vi "Transfer Count (Plugin).vi"(8 "error in (no error)":errorcluster, 11 "Plugin Configuration in":T1={"name"="", "components"=[], "cycle timing"={"priority"=0, "decimation"=1, "offset"=0}, "threads"=[], "Transfer Groups"=[], "settings"=[]} {"Transfer Groups"."Transfers"."channels"."string offset" format="%d bytes"}) -> (0 "error out":errorcluster, 2 "transfer count":i32, 3 "Plugin Configuration out":T1={"name"="", "components"=[], "cycle timing"={"priority"=0, "decimation"=1, "offset"=0}, "threads"=[], "Transfer Groups"=[], "settings"=[]} {"Transfer Groups"."Transfers"."channels"."string offset" format="%d bytes"})   [LabVIEW 2017, in "DSF Core.lvlib"]
uses:
  DSF Core.lvlib
  Controls/DSF Engine Plugin Configuration.ctl
  Controls/DSF Timing Info.ctl
  Controls/DSF Engine Plugin Thread Configuration.ctl
  Controls/DSF Settings Info.ctl
  Controls/DSF Engine Transfer Group Configuration.ctl
  Controls/DSF Direction.ctl
  Controls/DSF Engine Transfer Configuration.ctl
  Controls/DSF Byte Order.ctl
  Controls/DSF Engine Channel Configuration.ctl
  Controls/DSF Data Type.ctl
  Controls/DSF Timeout Behavior.ctl
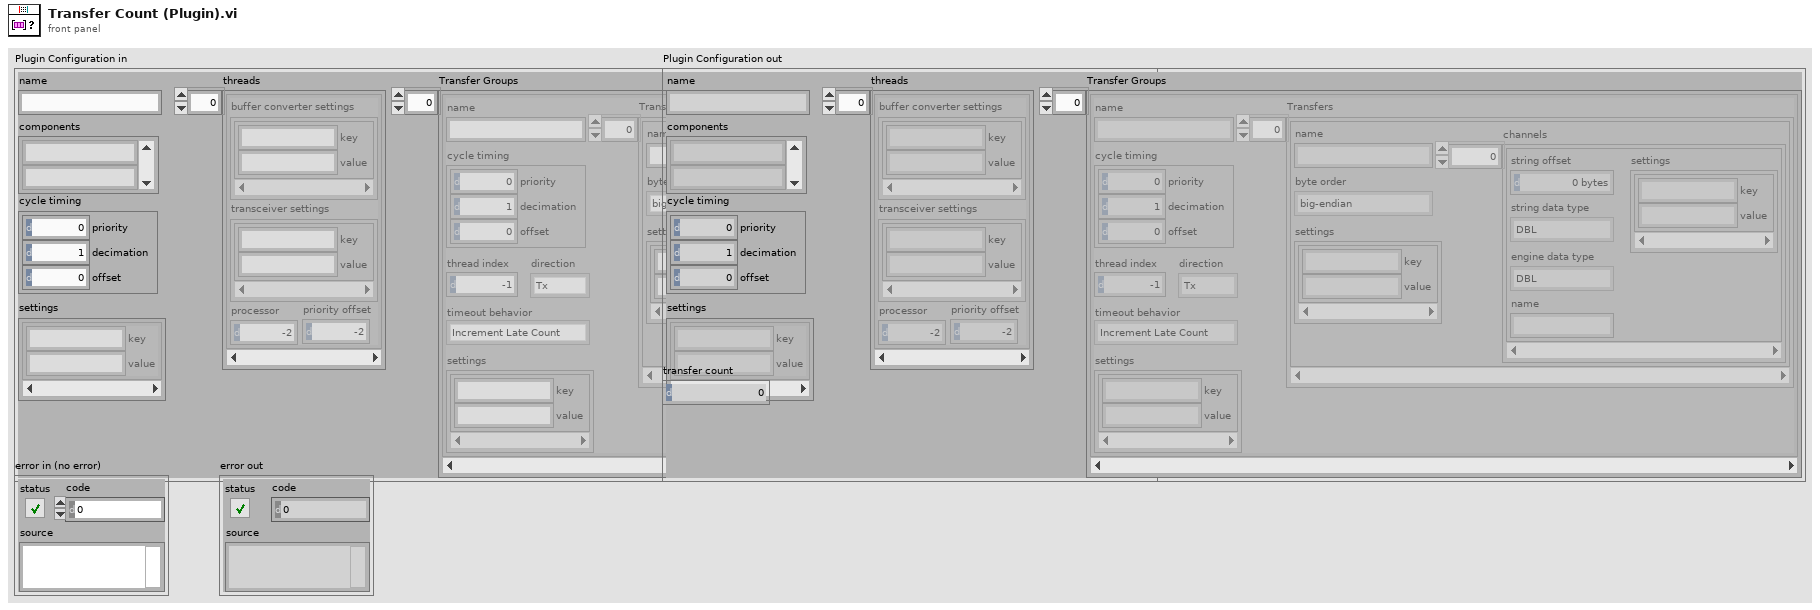
[diagram p1: front panel]
types:
  T1 = typedef "DSF Core.lvlib/DSF Engine Plugin Configuration.ctl" = cluster{"name":string, "components":string[], "cycle timing":T2, "threads":T3[], "Transfer Groups":T5[], "settings":T4}
  T2 = typedef "DSF Core.lvlib/DSF Timing Info.ctl" = cluster{"priority":u64, "decimation":u64, "offset":u64}
  T3 = typedef "DSF Core.lvlib/DSF Engine Plugin Thread Configuration.ctl" = cluster{"buffer converter settings":T4, "transceiver settings":T4, "processor":i32, "priority offset":i16}
  T4 = typedef "DSF Core.lvlib/DSF Settings Info.ctl" = cluster{"key":string, "value":string}[]
  T5 = typedef "DSF Core.lvlib/DSF Engine Transfer Group Configuration.ctl" = cluster{"name":string, "direction":T6, "cycle timing":T2, "thread index":i32, "settings":T4, "Transfers":T7[], "timeout behavior":T11}
  T6 = typedef "DSF Core.lvlib/DSF Direction.ctl" = enum8{"Tx", "Rx"}
  T7 = typedef "DSF Core.lvlib/DSF Engine Transfer Configuration.ctl" = cluster{"name":string, "byte order":T8, "settings":T4, "channels":T9[]}
  T8 = typedef "DSF Core.lvlib/DSF Byte Order.ctl" = enum8{"big-endian", "little-endian"}
  T9 = typedef "DSF Core.lvlib/DSF Engine Channel Configuration.ctl" = cluster{"string offset":u64, "string data type":T10, "engine data type":T10, "name":string, "settings":T4}
  T10 = typedef "DSF Core.lvlib/DSF Data Type.ctl" = enum8{"Bool", "SGL", "DBL", "I8", "I16", "I32", "I64", "U8", "U16", "U32", "U64"}
  T11 = typedef "DSF Core.lvlib/DSF Timeout Behavior.ctl" = enum8{"Increment Late Count", "Throw Error"}
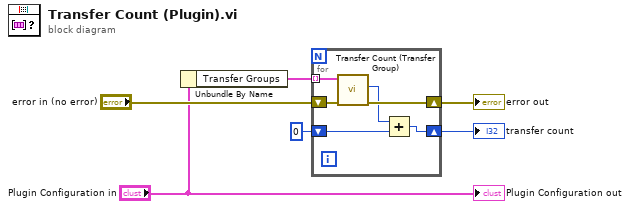
[diagram p0: block diagram]
diagram:
  n1 = Unbundle By Name("Plugin Configuration in") -> ("Transfer Groups"=w4:T5[])
  n2 = for {
    tunnel: w4 -> [w10] mode=indexing
    shift-right: [w12] -> w5
    shift-left: 0 -> [w11]
    shift-right: [w8] -> w3
    shift-left: "error in (no error)" -> [w9]
    n3 = call "Transfer Count (Transfer Group).vi"("error in (no error)"=w9, "Transfer Group Configuration in"=w10) -> ("error out"=w8:errorcluster, "transfer count"=w7:i32)  [unwired: 7 in, 1 out]
    n4 = Add(x=w7, y=w11) -> (x+y=w12:i32)
  }
  "transfer count" <- w5
  "error out" <- w3
  "Plugin Configuration out" <- "Plugin Configuration in"
